vi "Read test.vi"(8 "error in (no error)":errorcluster, 11 "Test Channel in":refnum<class "Test Channel.lvclass">) -> (0 "error out":errorcluster, 2 "test":dbl, 3 "Test Channel out":refnum<class "Test Channel.lvclass">)   [LabVIEW 2021, in "Test Channel.lvclass"]
uses:
  Test Channel.lvclass
  Test Channel.lvclass/Test Channel.ctl
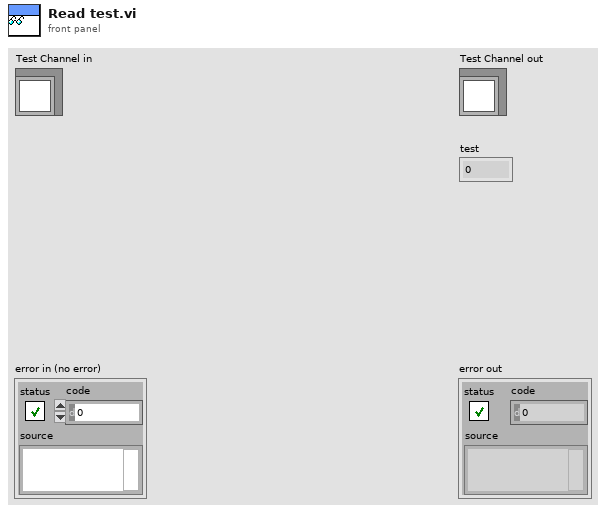
[diagram p1: front panel]
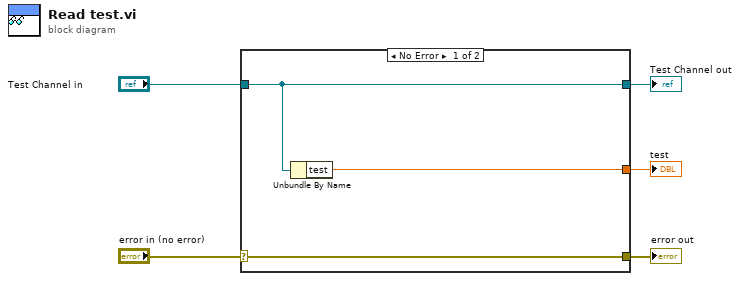
[diagram p0: block diagram]
diagram:
  n1 = case shown="No Error" "error in (no error)" {
    selector: "error in (no error)" -> [w8 w9]
    tunnel: [w8 w9] -> w4
    tunnel: [w7 w10] -> w2
    tunnel: "Test Channel in" -> [w7 w10]
    tunnel: [w6 _] -> w1
    frame No Error {
      n2 = Unbundle By Name(w7) -> ("test"=w6:dbl)
    }
    frame Error {
    }
  }
  "error out" <- w4
  "Test Channel out" <- w2
  "test" <- w1
